vi "Basic_Rewrite front panel name with running time of caller_8.5.vi"   [LabVIEW 2017, in "BasicVIs.lvlib"]
uses:
  BasicVIs.lvlib
panel:
  # "Change the caller's title to\n \n\"Last running time: XX/XX/XXXX XX:XX XX\" (Date and time) + original title"
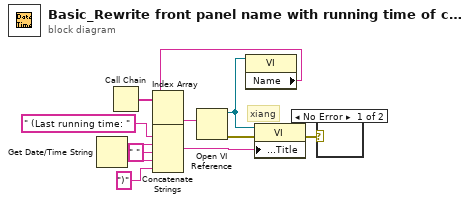
[diagram p0: block diagram]
diagram:
  # "xiang"
  n1 = Get Date/Time String() -> (date string=w11:string, time string=w9:string)  [unwired: 3 in]
  n2 = Call Chain() -> (call chain=w7:string[])
  n3 = Index Array(array=w7) -> (element #2=w6:string)  [unwired: 2 in, 1 out]
  n4 = Open VI Reference(vi path=w6) -> (vi reference=w2:refnum<vi>, error out=w5:errorcluster)  [unwired: 5 in]
  n5 = property class="VI"(reference=w2) -> ("Name"=w1:string)  [unwired: 1 in, 2 out]
  n6 = Concatenate Strings(w1, " (Last running time: " ("Label.Text"), w11, " " ("string"), w9, ")") -> (w10:string)
  n7 = property class="VI"(reference=w2, error in=w5, "Front Panel.Title"=w10) -> (error out=w4:errorcluster)  [unwired: 1 out]
  n8 = case shown="No Error" w4 {
    frame No Error {
    }
    frame Error {
    }
  }
